vi "ClearMessageControls.vi"(8 "error in (no error)":errorcluster, 11 "TCP_Client_Window in":refnum<class "TCP_Client_Window.lvclass">) -> (0 "error out":errorcluster, 3 "TCP_Client_Window out":refnum<class "TCP_Client_Window.lvclass">)   [LabVIEW 2023, in "TCP_Client_Window.lvlib" / "TCP_Client_Window.lvclass"]
uses:
  TCP_Client_Window.lvclass
  TCP_Client_Window.lvclass/TCP_Client_Window.ctl
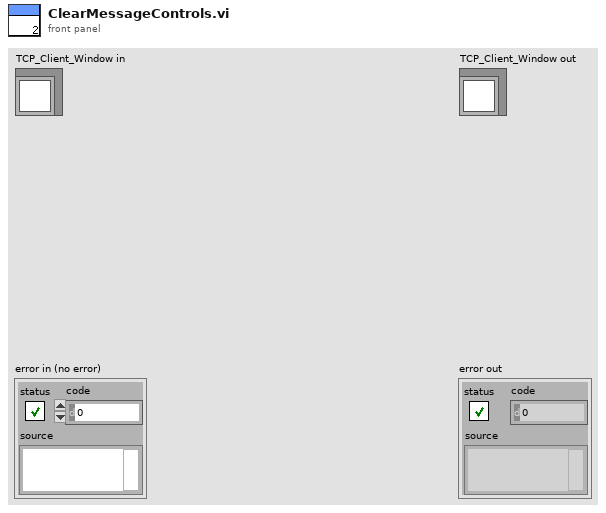
[diagram p1: front panel]
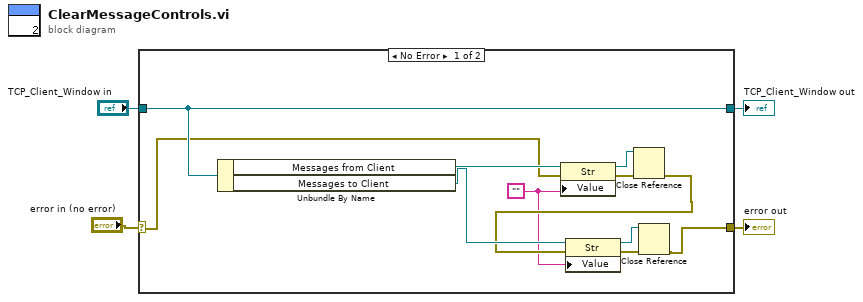
[diagram p0: block diagram]
diagram:
  n1 = case shown="No Error" "error in (no error)" {
    selector: "error in (no error)" -> [w8 w17]
    tunnel: [w6 w17] -> w3
    tunnel: [w15 w16] -> w1
    tunnel: "TCP_Client_Window in" -> [w15 w16]
    frame No Error {
      w5 = ""
      n2 = Unbundle By Name(w15) -> ("Messages from Client"=w10:refnum<vi>, "Messages to Client"=w9:refnum<vi>)
      n3 = property class="Str"(reference=w10, error in=w8, "Value"=w5) -> (reference out=w13:refnum<vi>, error out=w14:errorcluster)
      n4 = Close Reference(reference=w13, error in (no error)=w14) -> (error out=w7:errorcluster)
      n5 = property class="Str"(reference=w9, error in=w7, "Value"=w5) -> (reference out=w12:refnum<vi>, error out=w11:errorcluster)
      n6 = Close Reference(reference=w12, error in (no error)=w11) -> (error out=w6:errorcluster)
    }
    frame Error {
    }
  }
  "error out" <- w3
  "TCP_Client_Window out" <- w1
